vi "Check Library Name.vi"(8 "error in (no error)":errorcluster, 10 "Library Name":string) -> (0 "error out":errorcluster)   [LabVIEW 2020, in "WebServiceImporter.lvlib" / "Main Panel.lvlib" / "Input Info.lvlib"]
uses:
  <vilib>/Platform/WebService/Main Panel/Pages/Input Info/Input Info.lvlib
  <vilib>/Platform/WebService/Error Handling/Error/Error Number.ctl
  <vilib>/Platform/WebService/Error Handling/Error Handling.lvlib
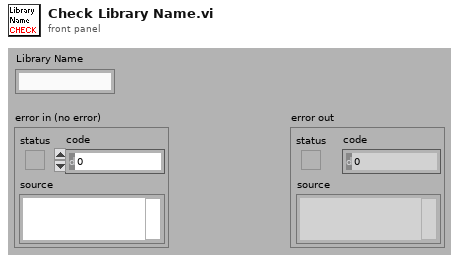
[diagram p1: front panel]
types:
  T1 = typedef "WebServiceImporter.lvlib/Error Handling.lvlib/Error Number.ctl" = u16
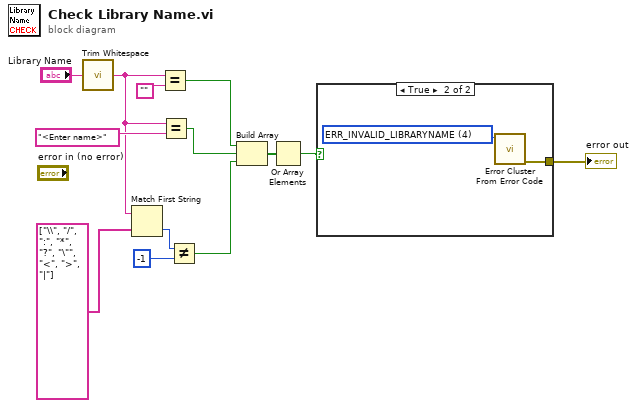
[diagram p0: block diagram]
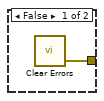
[diagram p2: hidden frame]
diagram:
  n1 = call <vilib>:"Trim Whitespace.vi"("string"="Library Name") -> ("trimmed string"=w8:string)  [unwired: 1 in]
  n2 = Match First String(2:string[] ["\\", "/", ":", "*", "?", "\"", "<", ">", "|"], 3:w8) -> (0:w2:i32)  [unwired: 1 out]
  n3 = Equal?(x=w8, y="") -> (x = y?=w6:bool)
  n4 = Equal?(x=w8, y="<Enter name>") -> (x = y?=w5:bool)
  n5 = Not Equal?(x=w2, y=-1) -> (x != y?=w1:bool)
  n6 = Build Array(w6, w5, w1) -> (w4:bool[])
  n7 = Or Array Elements(Boolean array=w4) -> (logical OR=w7:bool)
  n8 = case shown="True" w7 {
    tunnel: [w14 w15] -> w10
    frame False {
      n9 = call <vilib>:"Clear Errors.vi"() -> ("error out"=w14:errorcluster)  [unwired: 6 in, 1 out]
    }
    frame True {
      w16 = T1 4 items=["No Error", "ERR_INVALID_WSDL", "ERR_CREATE_PROXYDLL", "ERR_ACCESS_OUTPUTFOLDER", "ERR_INVALID_LIBRARYNAME"] ("Error Number")
      n10 = call <vilib>:"Error Cluster From Error Code.vi"("error code (0)"=w16) -> ("error out"=w15:errorcluster)  [unwired: 8 in]
    }
  }
  "error out" <- w10
